vi "niFPGALMRsmplLMOutSCTL.vi"(0 "input data":fxp<+/-,16,1>, 1 "reset":bool) -> (3 "channel index":u8, 4 "output data":fxp<+/-,18,1>, 10 "output valid":bool)   [LabVIEW 2017]
uses:
  <vilib>/Platform/TimedLoop/XDataNode/timing_clust.ctl
  <vilib>/Platform/TimedLoop/XDataNode/nitl_modes.ctl
  <vilib>/Platform/TimedLoop/XDataNode/wakeup.ctl
  <vilib>/Platform/TimedLoop/XDataNode/XDataNode.xnode
  <vilib>/Platform/TimedLoop/XDataNode/XDNodeRunTimeDep.lvlib
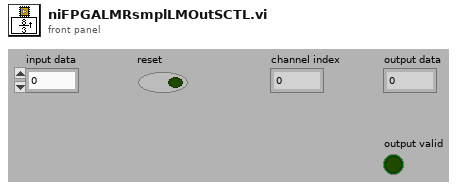
[diagram p1: front panel]
types:
  T1 = typedef "XDNodeRunTimeDep.lvlib/timing_clust.ctl" = cluster{"Expected End [f-1]":u64, "Actual End [f-1]":u64, "Finished Late? [f-1]":bool, "Expected End [i-1]":u64, "Actual End [i-1]":u64, "Finished Late? [i-1]":bool, "Expected Start [i]":u64, "Actual Start [i]":u64, "Expected Start [f]":u64, "Actual Start [f]":u64, "Source Name":string, "Structure Name":string, "Period":i64, "Deadline":i64, "Offset":i64, "Start":i64, "Priority":i32, "Timeout":i32, "Mode":T2, "Wakeup Reason":T3, "Error":errorcluster, "Source Type":string, "Secondary Source Type":string, "Global End Time":u64, "Global Start Time":u64, "Frame Duration":u64, "Iteration Duration":u64, "Assigned CPU":i32, "I/O Scan Engine Mode":u32}
  T2 = typedef "XDNodeRunTimeDep.lvlib/nitl_modes.ctl" = enum32{"No Change", "Process missed periods, maintain original phase", "Discard missed periods, maintain original phase", "Process missed periods, ignore original phase", "Discard missed periods, ignore original phase"}
  T3 = typedef "XDNodeRunTimeDep.lvlib/wakeup.ctl" = enum32{"Normal", "Aborted", "Asynchronous wakeup", "Timing source error", "Timed loop error", "Timeout"}
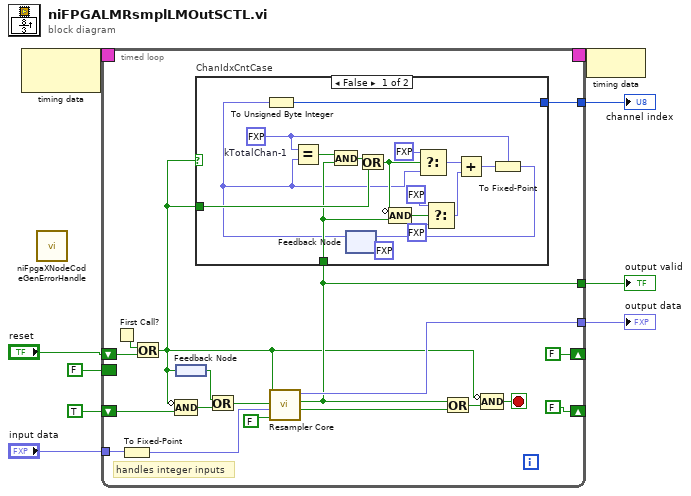
[diagram p0: block diagram]
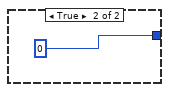
[diagram p2: hidden frame]
diagram:
  n1 = node-c288 ("Input Node")() -> (w9:T1)  [unwired: 1 out]
  n2 = call <vilib>:"niFpgaXNodeCodeGenErrorHandle.vi"() -> ()  [unwired: 1 in]
  n3 = timed-loop "Timed Loop" {
    timing: w9 -> [_]
    timing-out: [_] -> w8
    tunnel: "input data" -> [w14]
    tunnel: [w21] -> w7
    tunnel: [w23] -> w5
    shift-right: [FALSE] -> _
    shift-left: "reset" -> [w15]
    tunnel: [w25] -> w6
    shift-right: [FALSE] -> _
    shift-left: TRUE -> [w20]
    border: FALSE -> [_]
    stop <- w18 stop-if-true
    # "handles integer inputs"
    n4 = First Call?() -> (First Call?: T/F=w16:bool)
    n5 = To Fixed-Point(number=w14) -> (fixed-point=w13:fxp<+/-,16,1>)  [unwired: 1 in]
    n6 = Or(x=w16, y=w15) -> (x .or. y?=w11:bool)
    n7 = Compound Arithmetic op=AND(invert w11, w20) -> (w17:bool)
    n8 = feedback-in #1(w11) -> ()
    n9 = feedback #1() -> (w10:bool)
    n10 = Or(x=w10, y=w17) -> (x .or. y?=w12:bool)
    n11 = call "Resampler Core"("FIFOIsFull"=FALSE, "datain"=w13, "dataRDYIn"=w12, "reset"=w11) -> ("idle"=w22:bool, "dataRDYOut"=w21:bool, "y"=w23:fxp<+/-,18,1>)  [unwired: 5 in]
    n12 = case "ChanIdxCntCase" shown="False" w11 {
      tunnel: w11 -> [w42 _]
      tunnel: [w43 u8 0] -> w25
      tunnel: w21 -> [w40 _]
      frame False {
        w33 = fxp<+,1,1> 0.0  # kTotalChan-1
        n13 = feedback #2(fxp<+,1,1> 0.0) -> (w28:fxp<+,1,1>)
        n14 = To Unsigned Byte Integer(number=w28) -> (unsigned 8bit integer=w43:u8)
        n15 = Equal?(x=w33, y=w28) -> (x = y?=w41:bool)
        n16 = And(x=w41, y=w40) -> (x .and. y?=w39:bool)
        n17 = Or(x=w39, y=w42) -> (x .or. y?=w31:bool)
        n18 = Compound Arithmetic op=AND(invert w31, w40) -> (w30:bool)
        n19 = Select(t=fxp<+,1,1> 0.0 ("y"), s=w31, f=w28) -> (s? t:f=w37:fxp<+,1,1>)
        n20 = Select(t=fxp<+,1,1> 1.0 ("y"), s=w30, f=fxp<+,1,1> 0.0) -> (s? t:f=w35:fxp<+,1,1>)
        n21 = Add(x=w37, y=w35) -> (x+y=w34:fxp<+,2,2>)
        n22 = To Fixed-Point(fixed-point type=w33, number=w34) -> (fixed-point=w32:fxp<+,1,1>)
        n23 = feedback-in #2(w32) -> ()
      }
      frame True {
      }
    }
    n24 = Or(x=w21, y=w22) -> (x .or. y?=w19:bool)
    n25 = Compound Arithmetic op=AND(invert w11, w19) -> (w18:bool)
  }
  "channel index" <- w6
  "output valid" <- w7
  "output data" <- w5
  n26 = node-c288 ("Output Node")(w8) -> ()
